vi "Sensirion SHT25 - VISA I2C_USB command.vi"(7 "command":T1=1 items=["REVISION"=1, "NEW ADDRESS"=2, "SCAN1"=4, "SCAN2"=5, "SCAN3"=6, "SCAN4"=7, "SCAN6"=8, "SCAN8"=9, "SCAN12"=10, "SCAN16"=11, "SETPINS"=16, "GETPINS"=17, "GETAD"=18], 8 "Error In":errorcluster, 9 "data 2":string="\u0000", 10 "data 1":string="\u0000", 11 "VISA in":refnum<visa-resource-name>) -> (0 "Error Out":errorcluster, 1 "read buffer":string, 3 "VISA out":refnum<visa-resource-name>)   [LabVIEW 2012]
uses:
  Sensirion SHT25 - USB-I2C primary command.ctl
  Sensirion SHT25 - USB-I2C bytes returned.ctl
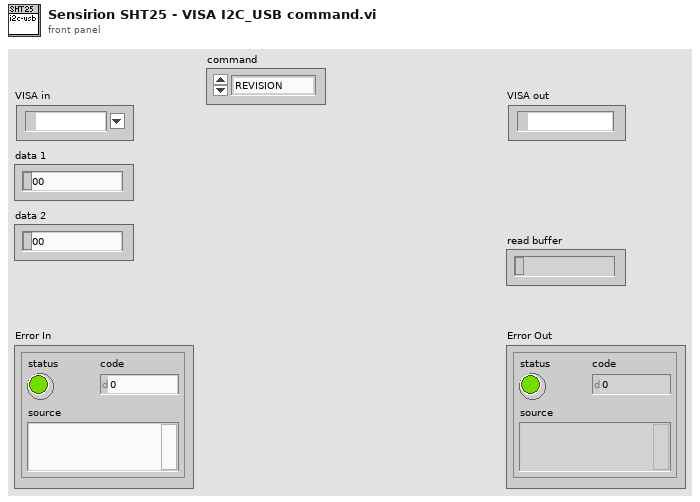
[diagram p1: front panel]
types:
  T1 = typedef "Sensirion SHT25 - USB-I2C primary command.ctl" = u8
  T2 = typedef "Sensirion SHT25 - USB-I2C bytes returned.ctl" = u32[]
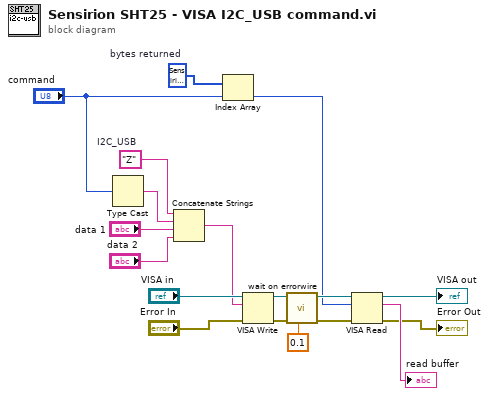
[diagram p0: block diagram]
diagram:
  w2 = T2 [0, 1, 1, 6, 6, 9, 12, 15, 21, 27, 39, 51, 0, 0, 0, 0, 1, 1, 4]  # bytes returned
  w5 = "Z"  # I2C_USB
  n1 = Type Cast(x="command") -> (*(type *) &x=w6:string)  [unwired: 1 in]
  n2 = Concatenate Strings(w5, w6, "data 1", "data 2") -> (w7:string)
  n3 = Index Array(array=w2, index="command") -> (element=w1:u32)
  n4 = VISA Write(VISA resource name="VISA in", write buffer=w7, error in (no error)="Error In") -> (VISA resource name out=w14:refnum<visa-resource-name>, error out=w16:errorcluster)  [unwired: 1 out]
  n5 = call "wait on errorwire.vi"("Delay Time (s)"=0.1, "error in (no error)"=w16) -> ("error out"=w13:errorcluster)  [unwired: 9 in]
  n6 = VISA Read(VISA resource name=w14, byte count=w1, error in (no error)=w13) -> (VISA resource name out=→"VISA out":refnum<visa-resource-name>, read buffer=→"read buffer":string, error out=→"Error Out":errorcluster)  [unwired: 1 out]
